vi "Track Previous Object.vi"(0 "Image_2d_u32 in":u32[][](array[numeric]) format="%08x", 5 "error in (no error)":errorcluster, 7 "Prev. Object Start/Stop/Sum":i32[][](array[numeric])) -> (11 "Col Offset":i32, 13 "Row Offset":i32, 14 "Image_2d_u32 out":u32[][](array[numeric]) format="%08x", 19 "error out":errorcluster)   [LabVIEW 2016]
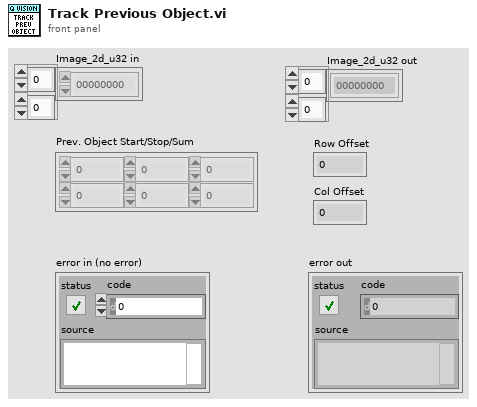
[diagram p1: front panel]
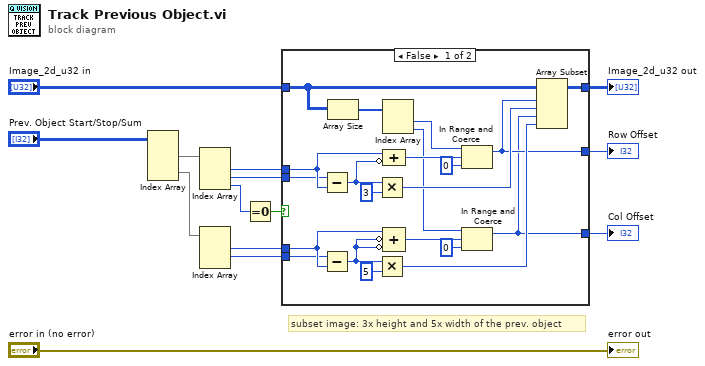
[diagram p0: block diagram]
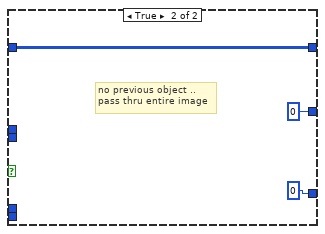
[diagram p2: hidden frame]
diagram:
  # "subset image: 3x height and 5x width of the prev. object"
  n1 = Index Array(array="Prev. Object Start/Stop/Sum") -> (element #1=w9:i32[], element #2=w1:i32[])  [unwired: 4 in]
  n2 = Index Array(array=w9) -> (element #1=w7:i32, element #2=w6:i32, element #3=w8:i32)  [unwired: 3 in]
  n3 = Index Array(array=w1) -> (element #1=w5:i32, element #2=w4:i32)  [unwired: 3 in, 1 out]
  n4 = Equal To 0?(x=w8) -> (x = 0?=w13:bool)
  n5 = case shown="False" w13 {
    tunnel: [w35 w38] -> w12
    tunnel: "Image_2d_u32 in" -> [w30 w38]
    tunnel: w7 -> [w34 _]
    tunnel: w6 -> [w32 _]
    tunnel: w5 -> [w21 _]
    tunnel: w4 -> [w20 _]
    tunnel: [w17 0 ("lower limit")] -> w3
    tunnel: [w16 0 ("lower limit")] -> w2
    frame False {
      n6 = Subtract(x=w32, y=w34) -> (x-y=w33:i32)
      n7 = Subtract(x=w20, y=w21) -> (x-y=w15:i32)
      n8 = Array Size(array=w30) -> (size(s)=w29:i32[])
      n9 = Multiply(x=w33, y=3) -> (x*y=w25:i32)
      n10 = Multiply(x=w15, y=5) -> (x*y=w18:i32)
      n11 = Index Array(array=w29) -> (element #1=w28:i32, element #2=w19:i32)  [unwired: 2 in]
      n12 = Compound Arithmetic op=ADD(w34, invert w33) -> (w27:i32)
      n13 = Compound Arithmetic op=ADD(w21, invert w15, invert w15) -> (w23:i32)
      n14 = In Range and Coerce(upper limit=w28, x=w27, lower limit=0) -> (coerced(x)=w17:i32)  [unwired: 1 out]
      n15 = In Range and Coerce(upper limit=w19, x=w23, lower limit=0) -> (coerced(x)=w16:i32)  [unwired: 1 out]
      n16 = Array Subset(array=w30, index (row)=w17, length (row)=w25, index (col)=w16, length (col)=w18) -> (w35:u32[][])
    }
    frame True {
      # "no previous object ..\npass thru entire image"
    }
  }
  "Image_2d_u32 out" <- w12
  "Row Offset" <- w3
  "Col Offset" <- w2
  "error out" <- "error in (no error)"
